vi "fromString.vi"(9 "DateTime String":string, 11 "DateTime.RFC5322 in":refnum<class "DateTime.RFC5322.lvclass">) -> (1 "Timestamp":timestamp, 3 "DateTime.RFC5322 out":refnum<class "DateTime.RFC5322.lvclass">)   [LabVIEW 2018, in "DateTime.RFC5322.lvclass"]
uses:
  <vilib>/LabVIEW Open Source Project/Epoch Date & Time/formatter.rfc5322/DateTime.RFC5322.lvclass
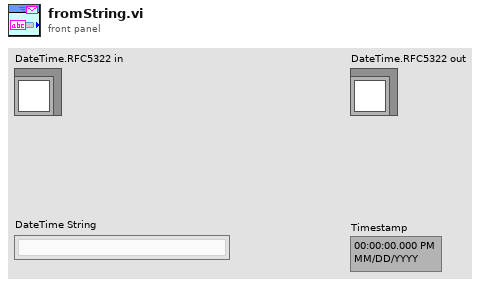
[diagram p1: front panel]
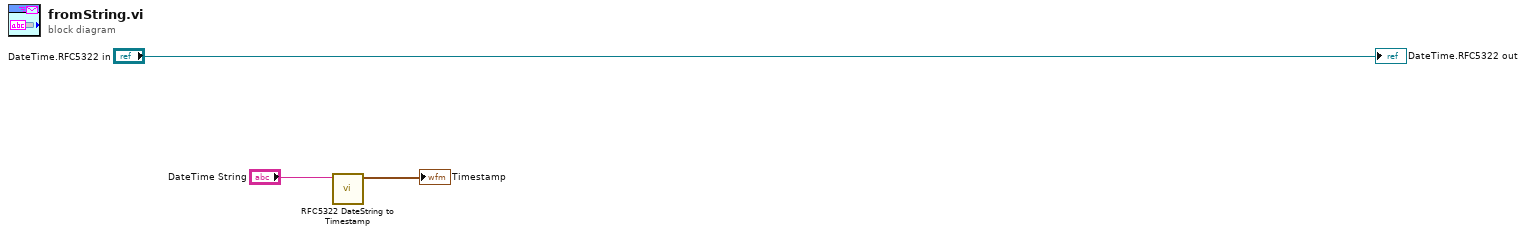
[diagram p0: block diagram]
diagram:
  n1 = call <vilib>:"RFC5322 DateString to Timestamp.vi"("RFC5322 Date String"="DateTime String") -> ("Timestamp"=→"Timestamp":timestamp)  [unwired: 8 in, 2 out]
  "DateTime.RFC5322 out" <- "DateTime.RFC5322 in"
